vi "FTW-Container-Support-XML-NodeType.vi"(0 "Element Node":refnum<k20>, 11 "error in":errorcluster) -> (4 "Element Node out":refnum<k20>, 6 "JSON Type":T1, 8 "Node XML Type":string, 15 "error out":errorcluster)   [LabVIEW 2012, in "FTW-Container.lvclass"]
uses:
  FTW-Container.lvclass
  JSON/FTW-JSON-Datatype.ctl
  <resource>/objmgr/DOMUserDefRef.rc
panel:
  # "Inputs"
  # "Outputs"
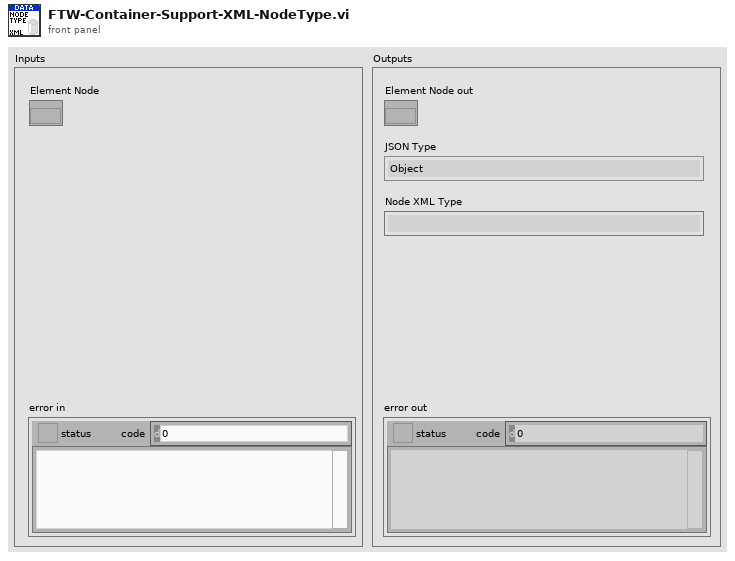
[diagram p1: front panel]
types:
  T1 = typedef "FTW-JSON-Datatype.ctl" = enum16{"Object", "Array", "String", "Number", "Boolean", "NULL", "<Refnum>", "<Enum>", "<Unknown>"}
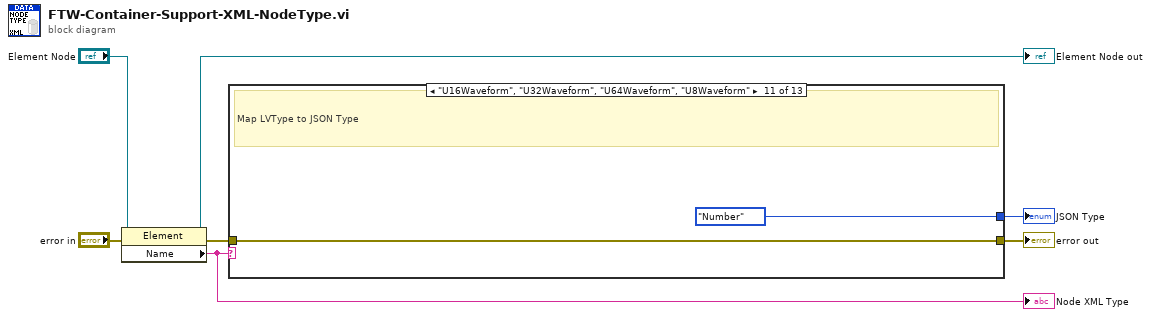
[diagram p0: block diagram]
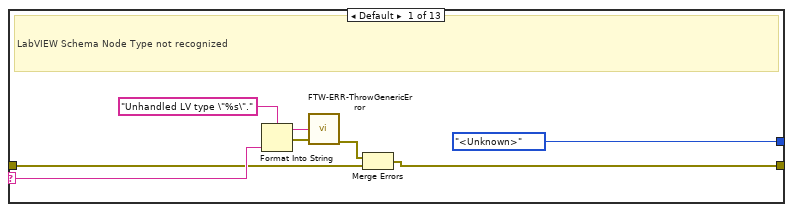
[diagram p2: hidden frame]
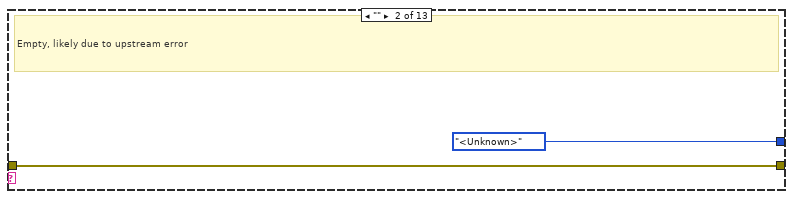
[diagram p3: hidden frame]
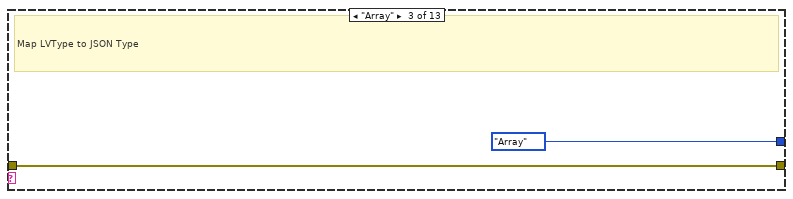
[diagram p4: hidden frame]
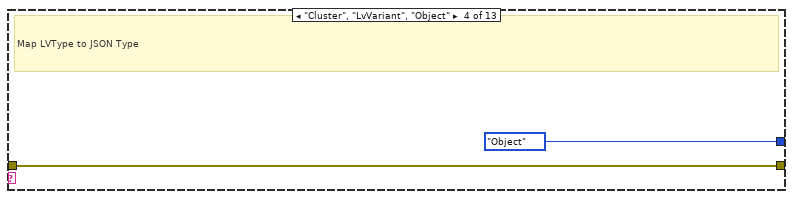
[diagram p5: hidden frame]
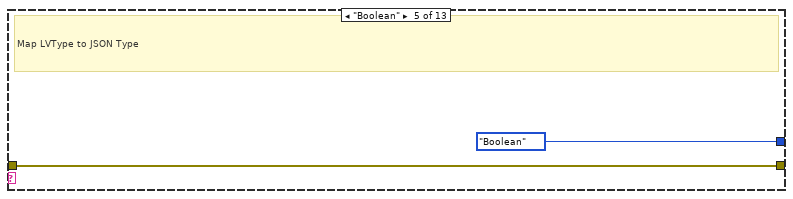
[diagram p6: hidden frame]
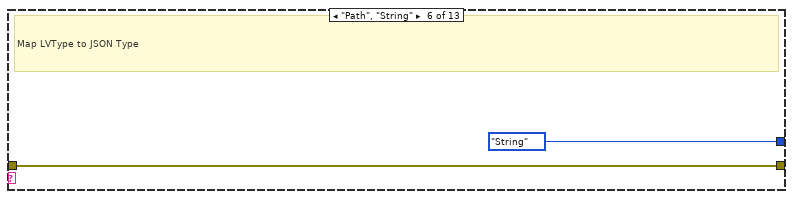
[diagram p7: hidden frame]
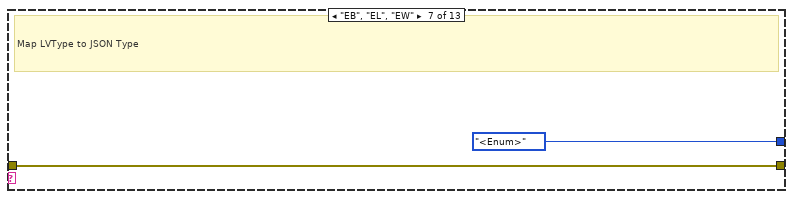
[diagram p8: hidden frame]
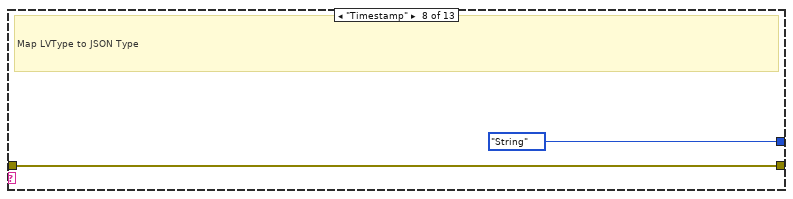
[diagram p9: hidden frame]
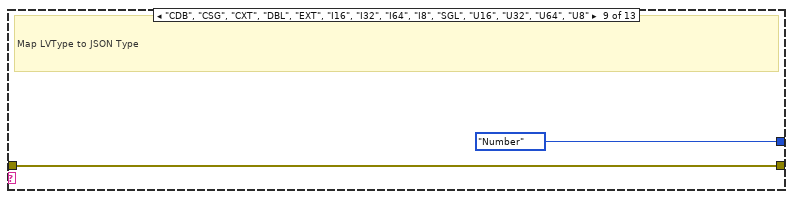
[diagram p10: hidden frame]
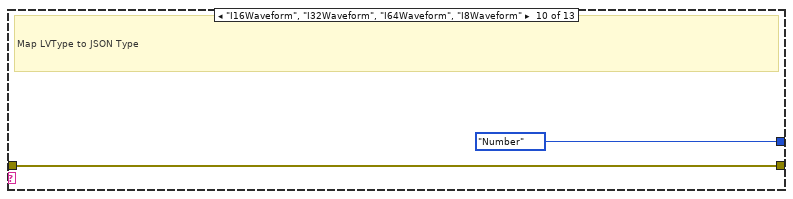
[diagram p11: hidden frame]
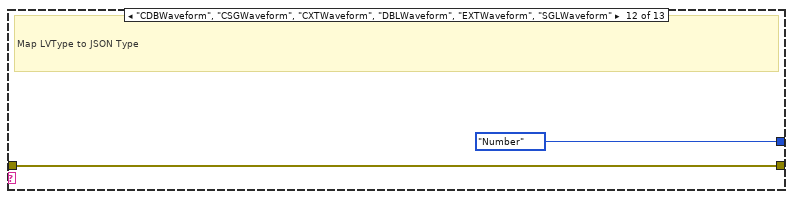
[diagram p12: hidden frame]
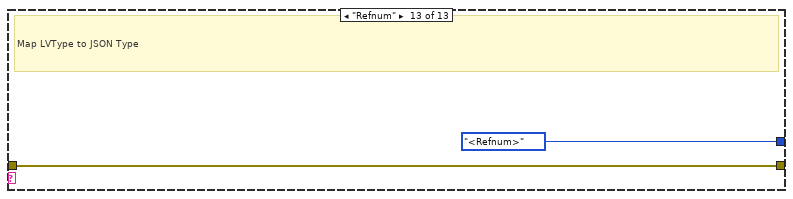
[diagram p13: hidden frame]
diagram:
  n1 = property class="Element"(reference="Element Node", error in="error in") -> (reference out=→"Element Node out":refnum<k20>, error out=w1:errorcluster, "Name"=w3:string)
  "Node XML Type" <- w3
  n2 = case shown="\"U16Waveform\", \"U32Waveform\", \"U64Waveform\", \"U8Waveform\"" w3 {
    selector: w3 -> [w14 _ _ _ _ _ _ _ _ _ _ _ _]
    tunnel: w1 -> [w11 w17 w19 w21 w23 w25 w27 w29 w31 w33 w35 w37 w39]
    tunnel: [FTW-JSON-Datatype."<Unknown>" ("JSON types") FTW-JSON-Datatype."<Unknown>" ("JSON types") FTW-JSON-Datatype."Array" ("JSON types") FTW-JSON-Datatype."Object" ("JSON types") FTW-JSON-Datatype."Boolean" ("JSON types") FTW-JSON-Datatype."String" ("JSON types") FTW-JSON-Datatype."<Enum>" ("JSON types") FTW-JSON-Datatype."String" ("JSON types") FTW-JSON-Datatype."Number" ("JSON types") FTW-JSON-Datatype."Number" ("JSON types") FTW-JSON-Datatype."Number" ("JSON types") FTW-JSON-Datatype."Number" ("JSON types") FTW-JSON-Datatype."<Refnum>" ("JSON types")] -> w2
    tunnel: [w10 w17 w19 w21 w23 w25 w27 w29 w31 w33 w35 w37 w39] -> w7
    frame Default {
      # "LabVIEW Schema Node Type not recognized"
      n3 = Format Into String(format string="Unhandled LV type \"%s\".", w14) -> (resulting string=w13:string, error out=w8:errorcluster)  [unwired: 2 in]
      n4 = call "FTW-ERR-ThrowGenericError.vi"("Error Message"=w13, "error in"=w8) -> ("error out"=w12:errorcluster)  [unwired: 13 in]
      n5 = Merge Errors(w12, w11) -> (w10:errorcluster)
    }
    frame "" {
      # "Empty, likely due to upstream error"
    }
    frame "Array" {
      # "Map LVType to JSON Type"
    }
    frame "Cluster", "LvVariant", "Object" {
      # "Map LVType to JSON Type"
    }
    frame "Boolean" {
      # "Map LVType to JSON Type"
    }
    frame "Path", "String" {
      # "Map LVType to JSON Type"
    }
    frame "EB", "EL", "EW" {
      # "Map LVType to JSON Type"
    }
    frame "Timestamp" {
      # "Map LVType to JSON Type"
    }
    frame "CDB", "CSG", "CXT", "DBL", "EXT", "I16", "I32", "I64", "I8", "SGL", "U16", "U32", "U64", "U8" {
      # "Map LVType to JSON Type"
    }
    frame "I16Waveform", "I32Waveform", "I64Waveform", "I8Waveform" {
      # "Map LVType to JSON Type"
    }
    frame "U16Waveform", "U32Waveform", "U64Waveform", "U8Waveform" {
      # "Map LVType to JSON Type"
    }
    frame "CDBWaveform", "CSGWaveform", "CXTWaveform", "DBLWaveform", "EXTWaveform", "SGLWaveform" {
      # "Map LVType to JSON Type"
    }
    frame "Refnum" {
      # "Map LVType to JSON Type"
    }
  }
  "error out" <- w7
  "JSON Type" <- w2
